vi "Read Mass.vi"(11 "Movable in":refnum<class "Movable.lvclass">) -> (2 "Mass":dbl)   [LabVIEW 2021, in "Movable.lvclass"]
doc: "MIT Licence\nCopyright (c) 2024 David Grollier"
uses:
  Movable.lvclass
  Movable.lvclass/Movable.ctl
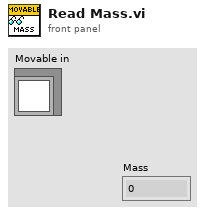
[diagram p1: front panel]
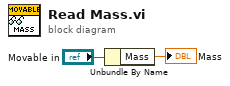
[diagram p0: block diagram]
diagram:
  n1 = Unbundle By Name("Movable in") -> ("Mass"=→"Mass":dbl)
